vi "picoscopeIndividualChannelSettings.vi"(11 "PicoscopeV2 in":refnum<class "PicoscopeV2.lvclass">) -> (3 "PicoscopeV2 out":refnum<class "PicoscopeV2.lvclass">)   [LabVIEW 2020, in "PicoscopeV2.lvclass"]
uses:
  PicoscopeV2.lvclass
  PicoscopeV2.lvclass/PicoscopeV2.ctl
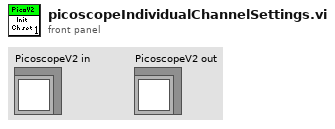
[diagram p1: front panel]
types:
  T1 = typedef "OnOffTypeDef.ctl" = enum16{"off", "on"}
  T2 = typedef "VoltageRange.ctl" = enum16{"10 mV", "20 mV", "50 mV", "100 mV", "200 mV", "500 mV", "1 V", "2 V", "5 V", "10 V", "20 V"}
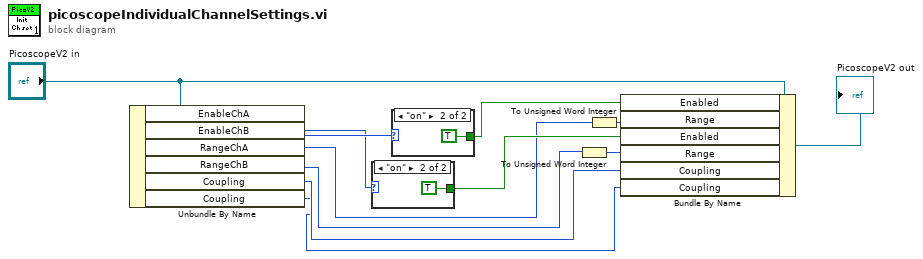
[diagram p0: block diagram]
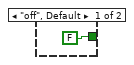
[diagram p2: hidden frame]
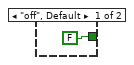
[diagram p3: hidden frame]
diagram:
  n1 = Unbundle By Name("PicoscopeV2 in") -> ("EnableChA"=w10:T1, "EnableChB"=w9:T1, "RangeChA"=w4:T2, "RangeChB"=w3:T2, "Coupling"=w2:i16, "Coupling"=w1:i16)
  n2 = case shown="\"on\"" w9 {
    tunnel: [FALSE TRUE] -> w7
    frame "off", Default {
    }
    frame "on" {
    }
  }
  n3 = case shown="\"on\"" w10 {
    tunnel: [FALSE TRUE] -> w8
    frame "off", Default {
    }
    frame "on" {
    }
  }
  n4 = To Unsigned Word Integer(number=w3) -> (unsigned 16bit integer=w5:u16)
  n5 = To Unsigned Word Integer(number=w4) -> (unsigned 16bit integer=w6:u16)
  n6 = Bundle By Name(cluster="PicoscopeV2 in", "Enabled"=w8, "Range"=w6, "Enabled"=w7, "Range"=w5, "Coupling"=w2, "Coupling"=w1) -> (→"PicoscopeV2 out":refnum<class "PicoscopeV2.lvclass">)
